vi "main_tb.vi"() -> ()   [LabVIEW 2018]
uses:
  Instrument/com.Instrument.lvlib
panel:
  in  "Emergency Stop":bool
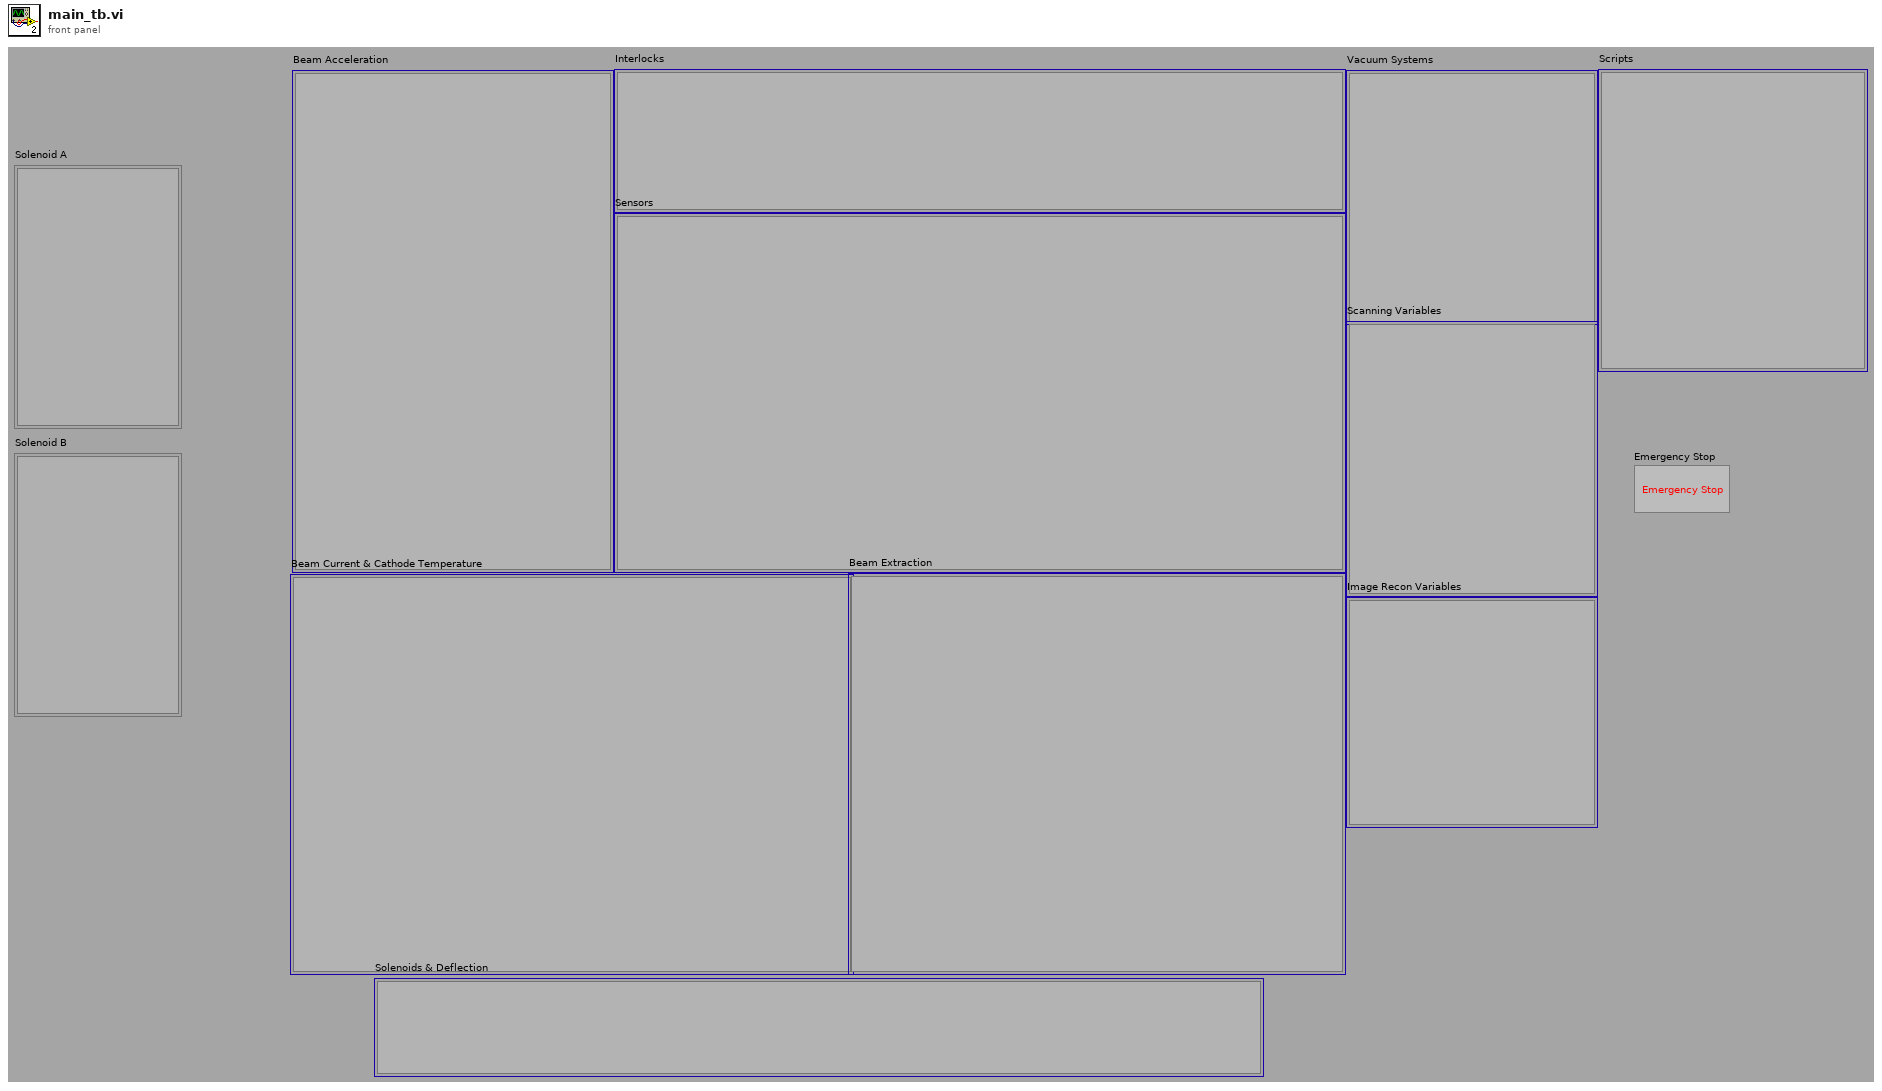
[diagram p1: front panel]
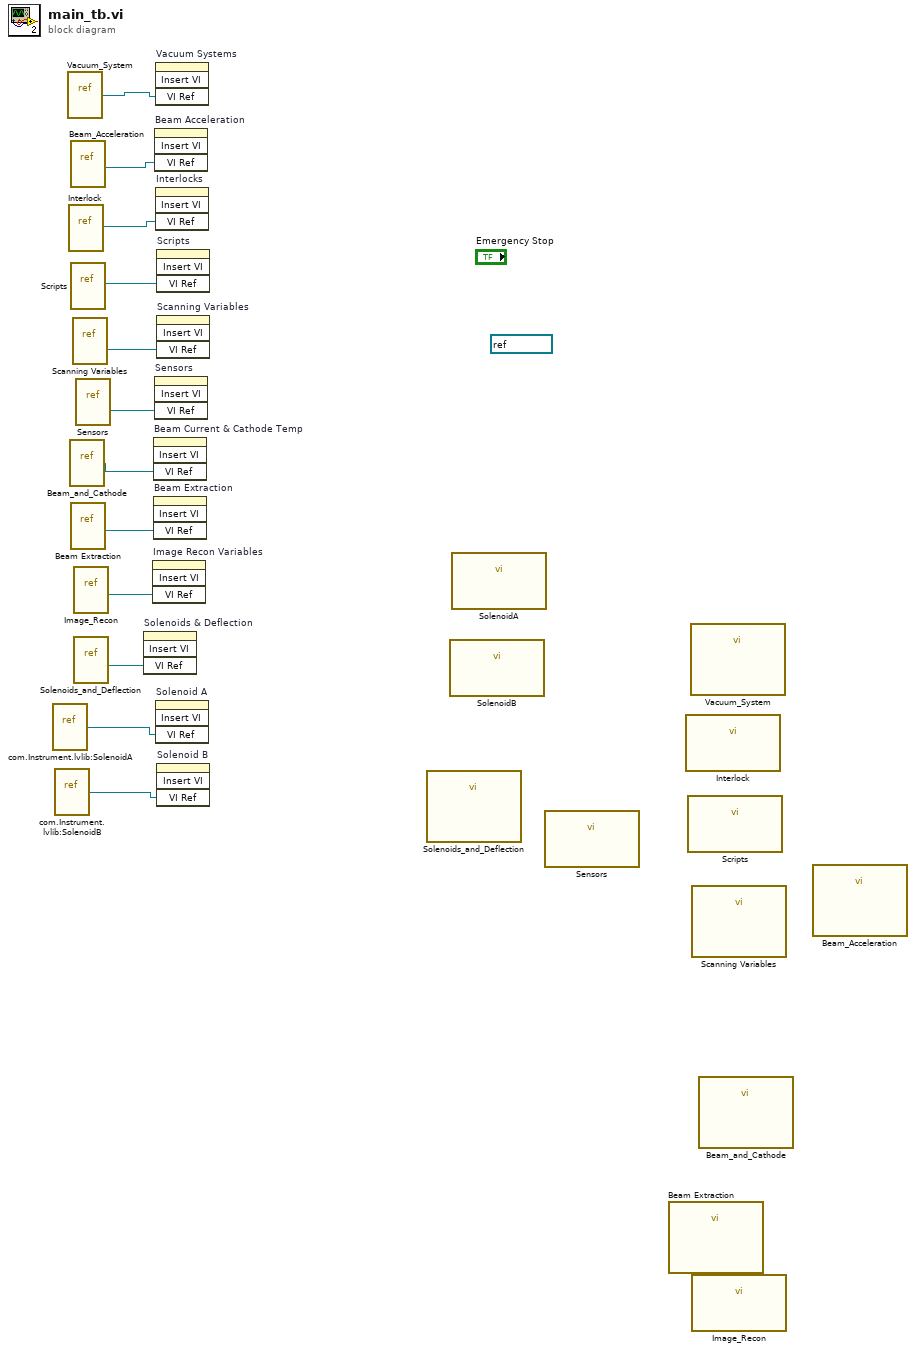
[diagram p0: block diagram]
diagram:
  (unwired) refnum<visa-resource-name> "COM1" ("VISA resource name")
  n1 = vi-ref "com.Instrument.lvlib:SolenoidA.vi"() -> (w2:refnum<vi>)
  n2 = vi-ref "com.Instrument.lvlib:SolenoidB.vi"() -> (w1:refnum<vi>)
  n3 = vi-ref "Vacuum_System.vi"() -> (w5:refnum<vi>)
  n4 = vi-ref "Interlock.vi"() -> (w10:refnum<vi>)
  n5 = vi-ref "Beam_and_Cathode.vi"() -> (w3:refnum<vi>)
  n6 = vi-ref "Beam_Acceleration.vi"() -> (w11:refnum<vi>)
  n7 = vi-ref "Scripts.vi"() -> (w9:refnum<vi>)
  n8 = vi-ref "Beam Extraction.vi"() -> (w12:refnum<vi>)
  n9 = vi-ref "Scanning Variables.vi"() -> (w8:refnum<vi>)
  n10 = vi-ref "Image_Recon.vi"() -> (w7:refnum<vi>)
  n11 = vi-ref "Solenoids_and_Deflection.vi"() -> (w6:refnum<vi>)
  n12 = vi-ref "Sensors.vi"() -> (w4:refnum<vi>)
  n13 = invoke on="Solenoids & Deflection" class="SubPnl" method="Insert VI"("VI Ref"=w6) -> ()  [unwired: 3 in, 4 out]
  n14 = invoke on="Image Recon Variables" class="SubPnl" method="Insert VI"("VI Ref"=w7) -> ()  [unwired: 3 in, 4 out]
  n15 = invoke on="Beam Current & Cathode Temp" class="SubPnl" method="Insert VI"("VI Ref"=w3) -> ()  [unwired: 3 in, 4 out]
  n16 = invoke on="Beam Extraction" class="SubPnl" method="Insert VI"("VI Ref"=w12) -> ()  [unwired: 3 in, 4 out]
  n17 = invoke on="Beam Acceleration" class="SubPnl" method="Insert VI"("VI Ref"=w11) -> ()  [unwired: 3 in, 4 out]
  n18 = invoke on="Sensors" class="SubPnl" method="Insert VI"("VI Ref"=w4) -> ()  [unwired: 3 in, 4 out]
  n19 = invoke on="Vacuum Systems" class="SubPnl" method="Insert VI"("VI Ref"=w5) -> ()  [unwired: 3 in, 4 out]
  n20 = invoke on="Interlocks" class="SubPnl" method="Insert VI"("VI Ref"=w10) -> ()  [unwired: 3 in, 4 out]
  n21 = invoke on="Solenoid A" class="SubPnl" method="Insert VI"("VI Ref"=w2) -> ()  [unwired: 3 in, 4 out]
  n22 = invoke on="Scripts" class="SubPnl" method="Insert VI"("VI Ref"=w9) -> ()  [unwired: 3 in, 4 out]
  n23 = invoke on="Scanning Variables" class="SubPnl" method="Insert VI"("VI Ref"=w8) -> ()  [unwired: 3 in, 4 out]
  n24 = invoke on="Solenoid B" class="SubPnl" method="Insert VI"("VI Ref"=w1) -> ()  [unwired: 3 in, 4 out]
  n25 = call "Solenoids_and_Deflection.vi"() -> ()  [unwired: 4 in]
  n26 = call "SolenoidB.vi"() -> ()  [unwired: 16 in]
  n27 = call "SolenoidA.vi"() -> ()  [unwired: 11 in]
  n28 = call "Sensors.vi"() -> ()  [unwired: 12 in]
  n29 = call "Beam Extraction.vi"() -> ()  [unwired: 12 in]
  n30 = call "Interlock.vi"() -> ()  [unwired: 12 in]
  n31 = call "Scripts.vi"() -> ()  [unwired: 12 in]
  n32 = call "Vacuum_System.vi"() -> ()  [unwired: 12 in]
  n33 = call "Scanning Variables.vi"() -> ()  [unwired: 12 in]
  n34 = call "Image_Recon.vi"() -> ()  [unwired: 12 in]
  n35 = call "Beam_and_Cathode.vi"() -> ()  [unwired: 12 in]
  n36 = call "Beam_Acceleration.vi"() -> ()  [unwired: 12 in]
